vi "Init.vi"(8 "error in (no error)":errorcluster, 11 "Mock In":refnum<class "Responsive Mock.lvclass">) -> (0 "error out":errorcluster, 3 "Mock Out":refnum<class "Responsive Mock.lvclass">)   [LabVIEW 2020, in "Responsive Mock.lvclass"]
uses:
  Responsive Mock.lvclass
  Expectation/Expectation.lvclass
  VI Call/VI Call.lvclass
  Responsive Mock.lvclass/Responsive Mock.ctl
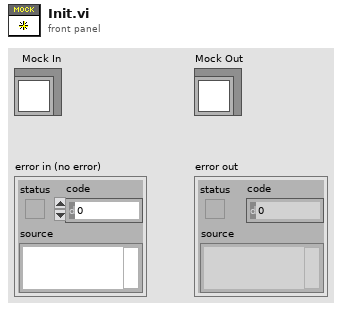
[diagram p1: front panel]
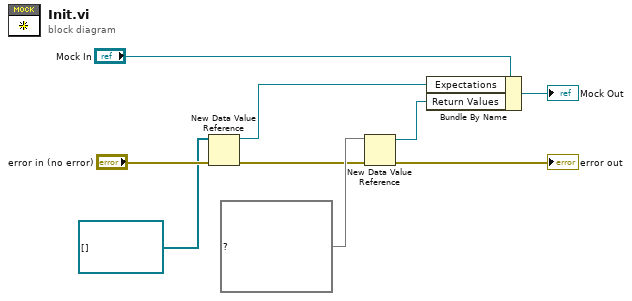
[diagram p0: block diagram]
diagram:
  n1 = New Data Value Reference(data value=refnum<class "Expectation.lvclass">[] [] ("Array"), error in="error in (no error)") -> (data value reference=w5:refnum<data-value>, error out=w3:errorcluster)
  n2 = New Data Value Reference(data value=map{string, refnum<queue>} {} ("Return Values 2"), error in=w3) -> (data value reference=w1:refnum<data-value>, error out=→"error out":errorcluster)
  n3 = Bundle By Name(cluster="Mock In", "Expectations"=w5, "Return Values"=w1) -> (→"Mock Out":refnum<class "Responsive Mock.lvclass">)
